vi "USRP Streaming to Memory FlexRIO (Host).vi"() -> ()   [LabVIEW 2016]
doc: "Example Description:\nStreams data through host memory from a RIO device then back to the RIO device at the specified rate(s).\n\nVI Configuration:\nThis example uses the PXI-7966R as the FPGA target by default. To use this VI with another FPGA target, use the following steps to configure the host VI to use a VI configured for your FPGA target:\n\n1. On the block diagram, right-click the Open FPGA VI Reference (PXI-7966R) VI and select Configure Open FPGA VI Reference.\n2. Browse for a new target by clicking the Browse Project button in the Open VI section.\n3. Select the VI under the target that matches your device. Click OK to select this VI.\n4. Click OK to exit the dialog box and to apply the new selection to the FPGA VI.\n\nRunning the VI:\n1. Select a RIO Resource that corresponds to the FPGA device configured above.\n2. Configure the Requested host Buffer Depth, Read/Write Size, and Requested (M) controls on the Host VI Front Panel.\n3. Click the run arrow to run the VI.\n4. Observe the Status of the Host Buffer as well as the Input and Output DMA FIFOs\n5. Observe the achieved Streaming Throughput.\n6. Click Stop on the Front Panel to stop the example\n\n\nExecution Steps:\nRefer to the block diagram of the Host VI for each example to view the execution steps for that specific example."
uses:
  <vilib>/userdefined/High Color/nirio_resource_hc.ctl
  <vilib>/FPGAPlugInAG/USRP 294xR; 295xR 200 MSps/niLvFpga_Open_USRP 294xR; 295xR 200 MSps.vi
  <vilib>/rvi/interface/common/dynamic/niFpgaDynamicAddResources.vi
  <vilib>/Utility/error.llb/Error Cluster From Error Code.vi
  <vilib>/rvi/errors/niLvFpgaAdjustHostInterfaceError.vi
  <vilib>/FPGAPlugInAG/Dynamic/niLvFpga_Run_Dynamic.vi
  <vilib>/rvi/interface/common/niFpgaWaitOnOcc.vi
  <vilib>/FPGAPlugInAG/Dynamic/niLvFpga_Close_Dynamic.vi
  <vilib>/rvi/interface/nirviOpenFPGA/nirviOpenFPGA.xnode
  Bitfiles/USRP-RIO-Streami_USRP294xR;295xR2_USRPThroughputSt_iEY1GQZeXEE.lvbitx
  <vilib>/rvi/interface/nirviReadWriteControl/nirviReadWriteControl.xnode
  <vilib>/rvi/interface/nirviMethod/nirviMethod.xnode
  <vilib>/rvi/interface/nirviCloseFPGA/nirviCloseFPGA.xnode
  <vilib>/rvi/interface/Simulation/niFpgaSimulationCallBeginRW.vi
  <vilib>/rvi/errors/niLvFpgaMergeErrorWithErrorCode.vi
  <vilib>/FPGAPlugInAG/Dynamic/niLvFpga_ConfigureFifo_Dynamic.vi
  <vilib>/FPGAPlugInAG/Dynamic/niLvFpga_StartFifo_Dynamic.vi
  <vilib>/FPGAPlugInAG/Dynamic/niLvFpga_AcquireReadRegionFifo_Dynamic.vi
  NiFpgaLv.dll
panel:
  in  "input.FIFO Size":u32
  out "error out":errorcluster
  in  "Stop":bool
  out "output.Host Buffer Status":cluster{u32, u32, u32}(slide) caption="Host Output Buffer Status" scale=0.0..67108864.0 scale format="%#.1p"
  out "input.Host Buffer Status":cluster{u32, u32, u32}(slide) caption="Host Input Buffer Status" scale=0.0..67108864.0 scale format="%#.1p"
  out "input.Host Buffer Depth (samples)":u32
  in  "Read/Write Size (samples)":u32=4194304 step=1048576
  in  "Requested Host Buffer Depth (samples)":u32=67108864 step=1048576
  in  "resource name":T1="Select RIO resource"
  out "input.Ever Timed Out?":bool caption="Overflow"
  in  "input.Reset":bool caption="Reset"
  out "input.FPGA FIFO Status":cluster{u32, u32}(slide) caption="FIFO Status" scale=0.0..65535.0 scale format="%#.1p"
  out "input.Max Throughput":u16 caption="Maximum (M)"
  in  "input.Requested Throughput":u16=1000 caption="Requested (M)" step=5
  out "input.Throughput (B/s)":dbl caption="Actual" format="%#.1p"
  out "Stop...":bool
  # "Configuration"
  # "Host"
  # "Input FPGA"
  # "Throughput (B/s)"
  # "Output FPGA"
  # "Throughput (B/s)"
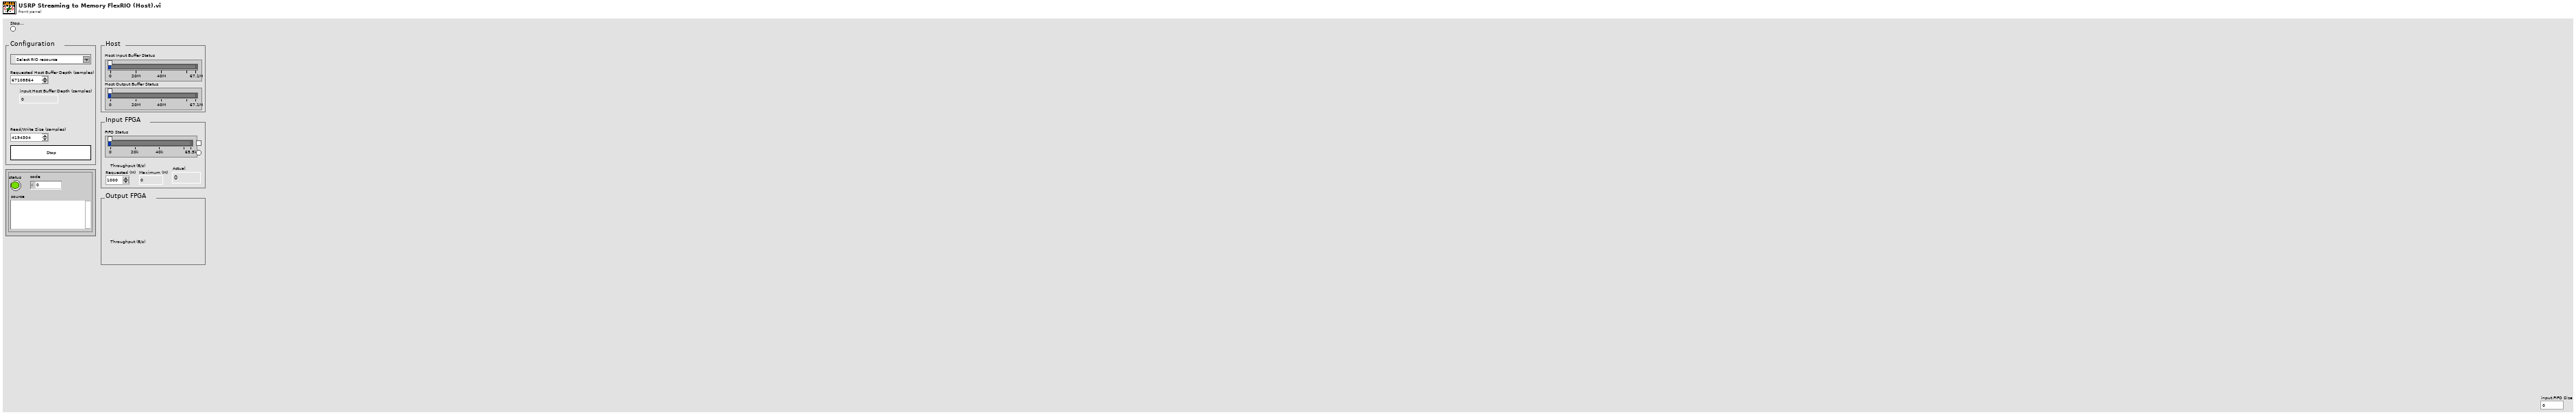
[diagram p1: front panel]
types:
  T1 = typedef "nirio_resource_hc.ctl" = tag
  T2 = cluster{"Iterations":u64, "Number of Elements Written":u64}
  T3 = cluster{"Current Amount Used":u32, "Maximum Amount Used":u32}
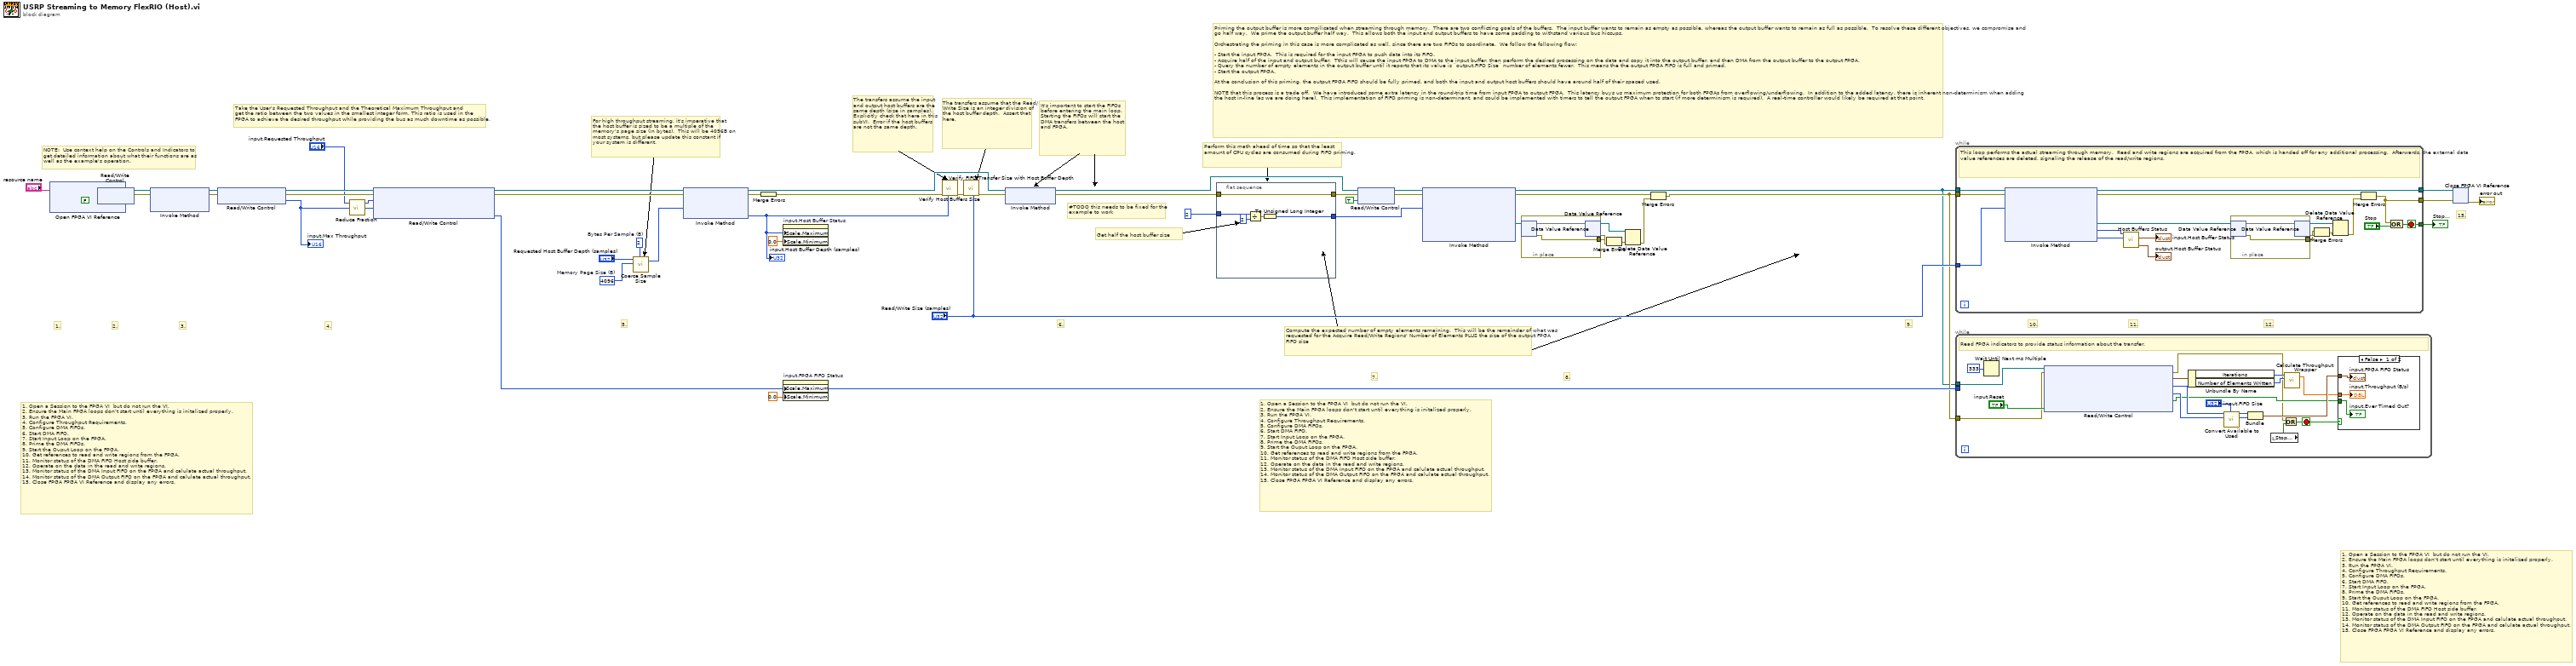
[diagram p0: block diagram]
diagram:
  w40 = u64 4096  # Memory Page Size (B)
  w42 = u64 2  # Bytes Per Sample (B)
  # "#TODO this needs to be fixed for the\nexample to work"
  # "1. Open a Session to the FPGA VI  but do not run the VI.\n2. Ensure the Main FPGA loops don't start until everything is initalized properly. \n3. Run the FPGA VI.\n4. Configure Throughput Requirements.\n5. Configure DMA FIFOs.\n6. Start DMA FIFO.\n7. Start Input Loop on the FPGA.\n8. Prime the DMA FIFOs.\n9. Start the Ouput Loop on the FPGA.\n10. Get references to read and write regions from the FPGA.\n11. Monitor status of the DMA FIFO Host side buffer.\n12. Operate on the data in the read and write regions. \n13. Monitor status of the DMA Input FIFO on the FPGA and calulate actual throughput.\n14. Monitor status of the DMA Output FIFO on the FPGA and calulate actual throughput.\n15. Close FPGA FPGA VI Reference and display any errors."
  # "1. Open a Session to the FPGA VI  but do not run the VI.\n2. Ensure the Main FPGA loops don't start until everything is initalized properly. \n3. Run the FPGA VI.\n4. Configure Throughput Requirements.\n5. Configure DMA FIFOs.\n6. Start DMA FIFO.\n7. Start Input Loop on the FPGA.\n8. Prime the DMA FIFOs.\n9. Start the Ouput Loop on the FPGA.\n10. Get references to read and write regions from the FPGA.\n11. Monitor status of the DMA FIFO Host side buffer.\n12. Operate on the data in the read and write regions. \n13. Monitor status of the DMA Input FIFO on the FPGA and calulate actual throughput.\n14. Monitor status of the DMA Output FIFO on the FPGA and calulate actual throughput.\n15. Close FPGA FPGA VI Reference and display any errors."
  # "12."
  # "10."
  # "15."
  # "Take the User's Requested Throughput and the Theoretical Maximum Throughput and\nget the ratio between the two values in the smallest integer form. This ratio is used in the \nFPGA to achieve the desired throughput while providing the bus as much downtime as possible."
  # "9."
  # "11."
  # "8."
  # "7."
  # "6."
  # "5."
  # "4."
  # "3."
  # "2."
  # "1. Open a Session to the FPGA VI  but do not run the VI.\n2. Ensure the Main FPGA loops don't start until everything is initalized properly. \n3. Run the FPGA VI.\n4. Configure Throughput Requirements.\n5. Configure DMA FIFOs.\n6. Start DMA FIFO.\n7. Start Input Loop on the FPGA.\n8. Prime the DMA FIFOs.\n9. Start the Ouput Loop on the FPGA.\n10. Get references to read and write regions from the FPGA.\n11. Monitor status of the DMA FIFO Host side buffer.\n12. Operate on the data in the read and write regions. \n13. Monitor status of the DMA Input FIFO on the FPGA and calulate actual throughput.\n14. Monitor status of the DMA Output FIFO on the FPGA and calulate actual throughput.\n15. Close FPGA FPGA VI Reference and display any errors."
  # "1."
  # "NOTE:  Use context help on the Controls and Indicators to \nget detailed information about what their functions are as\nwell as the example's operation."
  # "Compute the expected number of empty elements remaining.  This will be the remainder of what was requested for the Acquire Read/Write Regions' Number of Elements PLUS the size of the output FPGA FIFO size"
  # "Get half the host buffer size"
  # "Perform this math ahead of time so that the least amount of CPU cycles are consumed during FIFO priming."
  # "Priming the output buffer is more compilicated when streaming through memory.  There are two conflicting goals of the buffers.  The input buffer wants to remain as empty as possible, whereas the output buffer wants to remain as full as possible.  To resolve these different objectives, we compromise and go half way.  We prime the output buffer half way.  This allows both the input and output buffers to have some padding to withstand various bus hiccups.\n\nOrchestrating the priming in this case is more complicated as well, since there are two FIFOs to coordinate.  We follow the following flow:\n\n- Start the input FPGA.  This is required for the input FPGA to push data into its FIFO.\n- Acquire half of the input and output buffer.  Tthis will cause the input FPGA to DMA to the input buffer, then perform the desired processing on the data and copy it into the output buffer, and then DMA from the output buffer to the output FPGA.\n- Query the number of empty elements in the output buffer until it reports that its value is `output.FIFO Size` number of elements fewer.  This means the the output FPGA FIFO is full and primed.\n- Start the output FPGA.\n\nAt the conclusion of this priming, the output FPGA FIFO should be fully primed, and both the input and output host buffers should have around half of their spaced used.\n\nNOTE that this process is a trade off.  We have introduced some extra latency in the round-trip time from input FPGA to output FPGA.  This latency buys us maximum protection for both FPGAs from overflowing/underflowing.  In addition to the added latency, there is inherent non-determinism when adding the host in-line (as we are doing here).  This implementation of FIFO priming is non-determinant, and could be implemented with timers to tell the output FPGA when to start (if more determinism is required).  A real-time controller would likely be required at that point."
  # "For high throughput streaming, it's imperative that the host buffer is sized to be a multiple of the memory's page size (in bytes).  This will be 4096B on most systems, but please update this constant if your system is different."
  # "It's important to start the FIFOs before entering the main loop.  Starting the FIFOs will start the DMA transfers between the host and FPGA."
  # "The transfers assume that the Read/Write Size is an integer division of the host buffer depth.  Assert that here."
  # "The transfers assume the input and output host buffers are the same depth (size in samples).  Explicitly check that here in this subVI.  Error if the host buffers are not the same depth."
  n1 = xnode "Open FPGA VI Reference"("resource name"="resource name") -> ("FPGA VI Reference Out"=w49:refnum<k20>, "error out"=w48:errorcluster)  [unwired: 1 in]
  n2 = xnode "Read/Write Control"("FPGA VI Reference In"=w49, "error in"=w48, "input.Start"=FALSE) -> ("FPGA VI Reference Out"=w43:refnum<k20>, "error out"=w44:errorcluster)
  n3 = xnode "Invoke Method"("FPGA VI Reference In"=w43, "error in"=w44) -> ("FPGA VI Reference Out"=w27:refnum<k20>, "error out"=w26:errorcluster)  [unwired: 1 in]
  n4 = xnode "Read/Write Control"("FPGA VI Reference In"=w27, "error in"=w26) -> ("FPGA VI Reference Out"=w25:refnum<k20>, "error out"=w24:errorcluster, "input.Max Throughput"=w21:u16)
  "input.Max Throughput" <- w21
  n5 = call "Reduce Fraction.vi"("denominator"=w21, "numerator"="input.Requested Throughput") -> ("reduced denominator"=w23:u16, "reduced numerator"=w22:u16)  [unwired: 2 in]
  n6 = xnode "Read/Write Control"("FPGA VI Reference In"=w25, "error in"=w24, "input.Requested Throughput"=w22, "input.Requested Throughput Denominator"=w23) -> ("FPGA VI Reference Out"=w38:refnum<k20>, "error out"=w37:errorcluster, "input.FIFO Size"=w28:u32)
  n7 = call "Coerce Sample Size.vi"("Bytes Per Sample (B)"=w42, "Coerce To (B)"=w40, "Size (samples)"="Requested Host Buffer Depth (samples)") -> ("Coerced Size (samples)"=w36:u64)  [unwired: 4 in]
  n8 = xnode "Invoke Method"("FPGA VI Reference In"=w38, "error in"=w37, "Requested Depth"=w36) -> ("FPGA VI Reference Out"=w31:refnum<k20>, "error out"=w35:errorcluster, "Actual Depth"=w7:u32)
  "input.Host Buffer Depth (samples)" <- w7
  n9 = Merge Errors(w35) -> (w34:errorcluster)
  n10 = property on="input.Host Buffer Status" class="Slide (strict)"("Scale.Maximum"=w7, "Scale.Minimum"=0.0 ("Scale.Range:Minimum")) -> ()  [unwired: 2 in, 2 out]
  n11 = property on="input.FPGA FIFO Status" class="Slide (strict)"("Scale.Maximum"=w28, "Scale.Minimum"=0.0 ("Scale.Range:Minimum")) -> ()  [unwired: 2 in, 2 out]
  n12 = call "Verify Host Buffers Size.vi"("input.Host Buffer Size"=w7, "error in"=w34) -> ("error out"=w33:errorcluster)  [unwired: 9 in]
  n13 = call "Verify FIFO Transfer Size with Host Buffer Depth.vi"("Read/Write Size (samples)"="Read/Write Size (samples)", "error in"=w33) -> ("error out"=w30:errorcluster)  [unwired: 9 in]
  n14 = xnode "Invoke Method"("FPGA VI Reference In"=w31, "error in"=w30) -> ("FPGA VI Reference Out"=w1:refnum<k20>, "error out"=w2:errorcluster)
  n15 = flat-sequence {
    tunnel: u32 2 ("y") -> [w52]
    tunnel: [w54] -> w9
    tunnel: w2 -> [w53]
    tunnel: [w53] -> w8
    frame #0 {
      n16 = Divide(x=w52, y=u32 2) -> (x/y=w55:dbl)
      n17 = To Unsigned Long Integer(number=w55) -> (unsigned 32bit integer=w54:u32)
    }
  }
  n18 = xnode "Read/Write Control"("FPGA VI Reference In"=w1, "error in"=w8, "input.Start"=TRUE) -> ("FPGA VI Reference Out"=w18:refnum<k20>, "error out"=w17:errorcluster)
  n19 = xnode "Invoke Method"("FPGA VI Reference In"=w18, "error in"=w17, "Number of Elements"=w9) -> ("FPGA VI Reference Out"=w5:refnum<k20>, "error out"=w15:errorcluster, "Read Region Reference"=w16:refnum<data-value>)  [unwired: 1 in, 2 out]
  n20 = in-place {
    in-place-border: [w58] -> w11
    # "Insert additional processing here"
    n21 = in-place-dvr #1(w16) -> (w57:i16[], w58:errorcluster)
    n22 = in-place-dvr #1(w57) -> (w13:refnum<data-value>, w12:errorcluster)
  }
  n23 = Merge Errors(w11, w12) -> (w14:errorcluster)
  n24 = Delete Data Value Reference(data value reference=w13, error in=w14) -> (error out=w10:errorcluster)  [unwired: 1 out]
  n25 = Merge Errors(w15, w10) -> (w6:errorcluster)
  n26 = while {
    tunnel: w5 -> [w76]
    tunnel: w6 -> [w75]
    tunnel: "Read/Write Size (samples)" -> [w64]
    tunnel: [w72] -> w47
    tunnel: [w71] -> w45
    tunnel: [w69] -> w46
    stop <- w69 stop-if-true
    # "This loop performs the actual streaming through memory.  Read and write regions are acquired from the FPGA, which is handed off for any additional processing.  Afterwards, the external data value references are deleted, signaling the release of the read/write regions."
    n27 = xnode "Invoke Method"("FPGA VI Reference In"=w76, "error in"=w75, "Number of Elements"=w64) -> ("FPGA VI Reference Out"=w72:refnum<k20>, "error out"=w63:errorcluster, "Read Region Reference"=w74:refnum<data-value>, "Elements In Region"=w59:u32, "Elements Remaining"=w62:u32)  [unwired: 1 in]
    n28 = call "Host Buffers Status.vi"("input.Elements Remaining"=w62, "input.Elements In Region"=w59) -> ("output.Host Buffer Status"=→"output.Host Buffer Status":cluster{u32, u32, u32}, "input.Host Buffer Status"=→"input.Host Buffer Status":cluster{u32, u32, u32})  [unwired: 6 in, 2 out]
    n29 = in-place {
      in-place-border: [w78] -> w65
      # "Insert additional processing here"
      n30 = in-place-dvr #2(w74) -> (w77:i16[], w78:errorcluster)
      n31 = in-place-dvr #2(w77) -> (w68:refnum<data-value>, w66:errorcluster)
    }
    n32 = Merge Errors(w65, w66) -> (w67:errorcluster)
    n33 = Delete Data Value Reference(data value reference=w68, error in=w67) -> (error out=w73:errorcluster)  [unwired: 1 out]
    n34 = Merge Errors(w63, w73) -> (w71:errorcluster)
    n35 = Compound Arithmetic op=OR(w71, "Stop") -> (w69:bool)
  }
  "Stop..." <- w46
  n36 = while {
    tunnel: w6 -> [w80]
    tunnel: w28 -> [_]
    tunnel: w5 -> [w81]
    stop <- w94 stop-if-true
    # "Read FPGA indicators to provide status information about the transfer."
    n37 = Wait Until Next ms Multiple(millisecond multiple=u32 333) -> ()  [unwired: 1 out]
    n38 = xnode "Read/Write Control"("FPGA VI Reference In"=w81, "error in"=w80, "input.Reset"="input.Reset") -> ("error out"=w79:errorcluster, "input.FIFO Transfer Status"=w93:T2, "input.Number of Elements to Write"=w86:u32, "input.Minimum Number of Elements to Write"=w87:u32, "input.Ever Timed Out?"=w83:bool)  [unwired: 1 out]
    n39 = Unbundle By Name(w93) -> ("Iterations"=w91:u64, "Number of Elements Written"=w92:u64)
    n40 = call "Convert Available to Used.vi"("Size"="input.FIFO Size", "Minimum Amount Available"=w87, "Current Amount Available"=w86) -> ("Maximum Amount Used"=w89:u32, "Current Amount Used"=w88:u32)  [unwired: 5 in]
    n41 = Bundle("Current Amount Used"=w88, "Maximum Amount Used"=w89) -> (w85:T3)  [unwired: 1 in]
    n42 = local read "Stop..."() -> (w95:bool)
    n43 = Or(x=w79, y=w95) -> (x .or. y?=w94:bool)
    n44 = call "Calculate Throughput Wrapper.vi"("transfers"=w92, "iterations"=w91) -> ("throughput (B/s)"=w84:dbl)  [unwired: 3 in]
    n45 = case shown="False" w94 {
      tunnel: w85 -> [w99 _]
      tunnel: w84 -> [w98 _]
      tunnel: w83 -> [w97 _]
      frame False {
        "input.Throughput (B/s)" <- w98
        "input.Ever Timed Out?" <- w97
        "input.FPGA FIFO Status" <- w99
      }
      frame True {
      }
    }
  }
  n46 = xnode "Close FPGA VI Reference"("FPGA VI Reference In"=w47, "error in"=w45) -> ("error out"=→"error out":errorcluster)
